vi "FTW-CodeGen-GenerateCode.vi"(0 "State In":T2, 5 "XRef":refnum<vi>, 7 "Terms":T1(array[cluster]), 9 "Diagram":refnum<vi>) -> (4 "State Out":T2, 6 "Reply":string[](array[string]), 8 "Generated Code?":bool)   [LabVIEW 2015, in "FTW-SQLite-Insert.xnode"]
uses:
  FTW-SQLite-Insert.xnode
  FTW-CodeGen-State.ctl
  FTW-CodeGen-XNodeCommonState.ctl
  FTW-CodeGen-XNodeReplyType.ctl
panel:
  # "Inputs"
  # "Outputs"
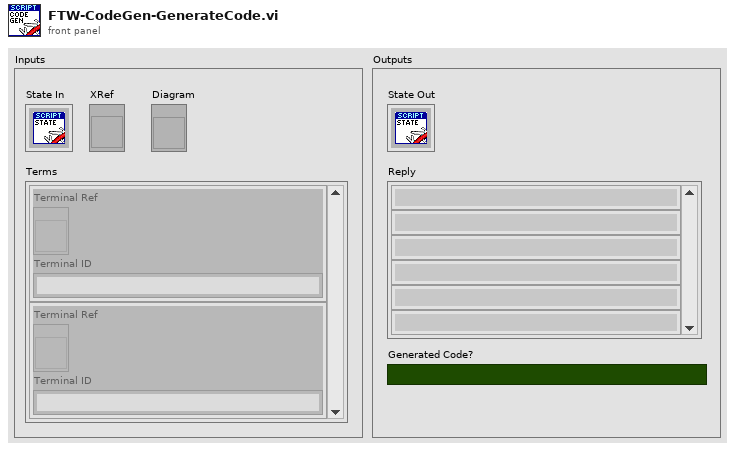
[diagram p1: front panel]
types:
  T1 = cluster{"Terminal Ref":refnum<vi>, "Terminal ID":string}[]
  T2 = typedef "FTW-SQLite-Insert.xnode/FTW-CodeGen-State.ctl" = cluster{"Cache":T3}
  T3 = typedef "FTW-CodeGen-XNodeCommonState.ctl" = cluster{"Terms":cluster{"Name":string, "Id":string, "Type":variant, "Bounds":cluster{"Left":i32, "Top":i32, "Right":i32, "Bottom":i32}, "Input?":bool, "Required?":bool, "Recommended?":bool, "Adaptive?":bool, "Hidden?":bool, "Direction":enum32{"Auto", "Up", "Down", "Left", "Right", "Center"}, "Break Wire?":bool, "English Name":string}[], "AdaptiveTerms":string[], "AdaptedTypes":variant[], "ForceCodeRegeneration?":bool, "LastGeneration":timestamp, "Errors":string[]}
  T4 = typedef "FTW-CodeGen-XNodeReplyType.ctl" = enum16{"UpdateState", "AdaptToInputs", "AdaptAndAugment", "CosmeticUpdate", "NoReply"}
  T5 = typedef "FTW-Reflection-Types.ctl" = enum16{"Unknown", "Void", "Array", "Cluster", "LVObject", "Boolean", "I8", "I16", "I32", "I64", "U8", "U16", "U32", "U64", "SGL", "DBL", "EXT", "CSG", "CDB", "CXT", "FXP", "EnumU8", "EnumU16", "EnumU32", "EnumU64", "SGLwithUnit", "DBLwithUnit", "EXTwithUnit", "CSGwithUnit", "CDBwithUnit", "CXTwithUnit", "String", "Path", "Picture", "Tag", "LVVariant", "Timestamp", "WaveformI8", "WaveformI16", "WaveformI32", "WaveformI64", "WaveformU8", "WaveformU16", "WaveformU32", "WaveformU64", "WaveformSGL", "WaveformDBL", "WaveformEXT", "WaveformCSG", "WaveformCDB", "WaveformCXT", "WaveformDigital", "WaveformUnknownType", "DigitalData", "DynamicData", "ExternalData", "FileByteStream", "TDMStream", "dotNET", "ActiveX", "VIServerReference", "VIReference", "ApplicationInstance", "Menu", "ConnectionDataSocket", "ConnectionVISA", "ConnectionBluetooth", "ConnectionIrDA", "ConnectionTCP", "ConnectionUDP", "ConnectionHTTPClient", "ConnectionFTP", "Occurrence", "Notifier", "Queue", "Rendezvous", "Semaphore", "RTFIFO", "EventPublisher", "EventRegistration", "EventCallback", "DataValueReference", "GenericClass", "GenericClassTag", "GenericClassDeepCopy", "GenericClassFlattened", "GenericClassTagFlattened", "GenericReferenceType", "WindowsRegistry", "OverloadedDatalogRef", "ReferenceUnknownType", "ByteArray", "ConPaneInterface", "FTWObject"}
  T6 = cluster{"Element Name":string, "Element Type":T5, "Element Value":variant}[]
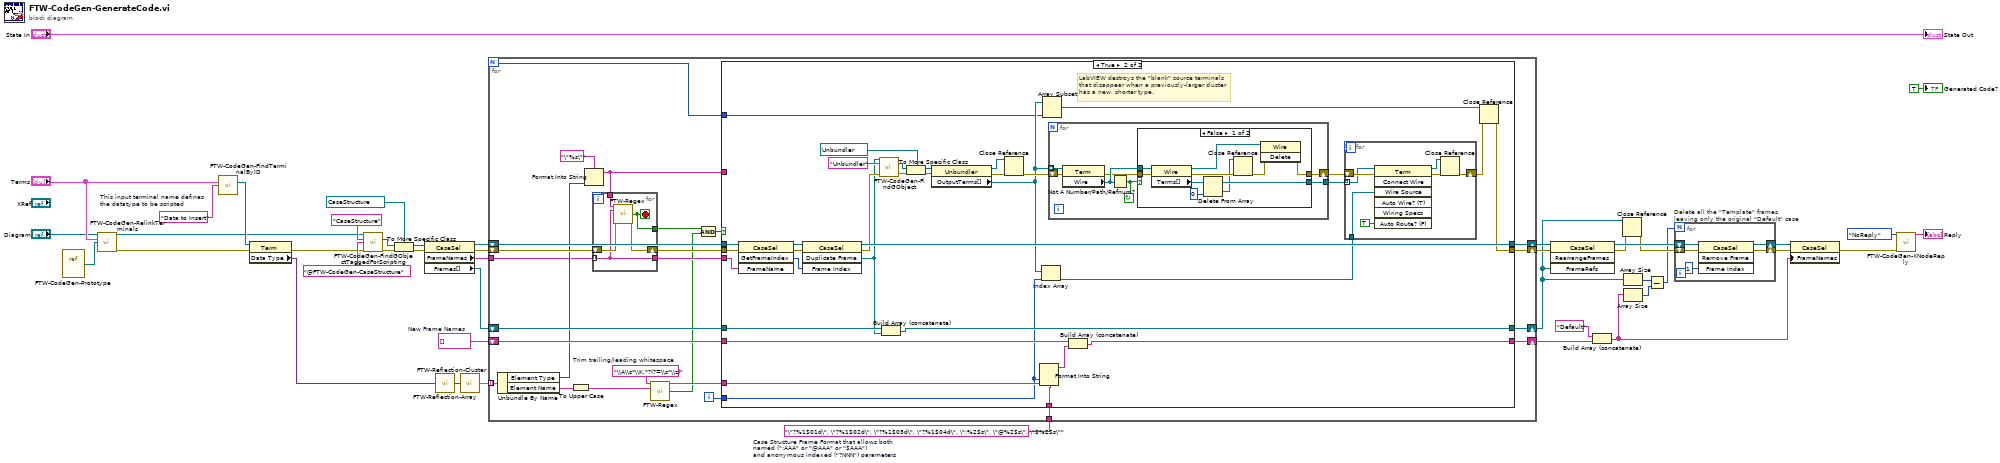
[diagram p0: block diagram]
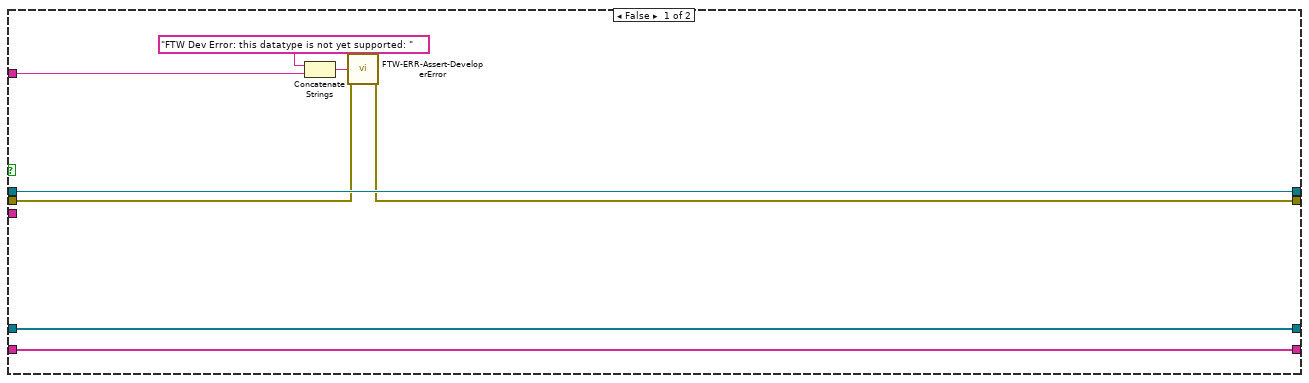
[diagram p2: hidden frame]
diagram:
  w13 = "\"?%1$01d\", \"?%1$02d\", \"?%1$03d\", \"?%1$04d\", \":%2$s\", \"@%2$s\", \"$%2$s\""  # Case Structure Frame Format that allows both named (":AAA" or "@AAA" or "$AAA") and anonymous indexed ("?NNN") parameters
  w1 = string[] []  # New Frame Names
  w4 = "Data to Insert"  # This input terminal name defines the datatype to be scripted
  n1 = vi-ref "FTW-CodeGen-Prototype.vi"() -> (w7:refnum<vi>)
  n2 = call "FTW-CodeGen-RelinkTerminals.vi"("Diagram"="Diagram", "Terms"="Terms", "PrototypeVI"=w7) -> ("Diagram out"=w2:refnum<vi>, "error out"=w10:errorcluster)  [unwired: 11 in]
  n3 = call "FTW-CodeGen-FindTerminalByID.vi"("Terms"="Terms", "Terminal ID"=w4) -> ("Terminal Ref"=w6:refnum<vi>)  [unwired: 12 in, 1 out]
  n4 = property class="Term"(reference=w6, error in=w10) -> (error out=w9:errorcluster, "Data Type"=w15:variant)  [unwired: 1 out]
  n5 = call "FTW-CodeGen-FindGObjectTaggedForScripting.vi"("GObject to Traverse"=w2, "Class Name"="CaseStructure", "Label Prefix to uniquely identify node"="@FTW-CodeGen-CaseStructure" ("Label to uniquely identify node"), "error in"=w9) -> ("GObject"=w40:refnum<vi>, "error out"=w39:errorcluster)  [unwired: 9 in, 1 out]
  n6 = To More Specific Class(target class=refnum<vi> refnum ("Object"), reference=w40, error in=w39) -> (specific class reference=w36:refnum<vi>, error out=w34:errorcluster)
  n7 = property class="CaseSel"(reference=w36, error in=w34) -> (reference out=w35:refnum<vi>, error out=w33:errorcluster, "FrameNames"=w32:string[], "Frames[]"=w21:refnum<vi>[])
  n8 = call "FTW-Reflection-Array.vi"("Array"=w15) -> ("Default Array Element"=w14:variant)  [unwired: 13 in, 1 out]
  n9 = call "FTW-Reflection-Cluster.vi"("Cluster"=w14) -> ("Cluster Elements"=w37:T6)  [unwired: 14 in]
  n10 = for {
    N -> [w44]
    tunnel: w37 -> [w66] mode=indexing
    tunnel: w32 -> [w52]
    shift-right: [w61] -> w26
    shift-left: w35 -> [w68]
    shift-right: [w62] -> w24
    shift-left: w33 -> [w67]
    shift-right: [w60] -> w20
    shift-left: w21 -> [w63]
    shift-right: [w58] -> w27
    shift-left: w1 -> [w59]
    tunnel: w13 -> [w54]
    i -> [w55]
    w48 = "\\A\\s*\\K.*?(?=\\s*\\z)"  # Trim trailing/leading whitespace
    n11 = Unbundle By Name(w66) -> ("Element Type"=w56:T5, "Element Name"=w57:string)
    n12 = To Upper Case(1:w57) -> (0:w50:string)
    n13 = Format Into String(format string="\"%s\"", w56) -> (resulting string=w64:string)  [unwired: 2 in, 1 out]
    n14 = for {
      tunnel: w64 -> [w72]
      shift-right: [w71] -> w53
      shift-left: w67 -> [w73]
      tunnel: w52 -> [w69] mode=indexing
      tunnel: [w70] -> w47
      tunnel: [w69] -> w51
      stop <- w70 stop-if-true
      n15 = call "FTW-Regex.vi"("Regular Expression"=w72, "Input String"=w69, "error in"=w73) -> ("Match Found?"=w70:bool, "error out"=w71:errorcluster)  [unwired: 8 in, 3 out]
    }
    n16 = call "FTW-Regex.vi"("Regular Expression"=w48, "Input String"=w50) -> ("Match"=w49:string, "Match Found?"=w45:bool)  [unwired: 9 in, 3 out]
    n17 = Compound Arithmetic op=AND(w47, w45) -> (w46:bool)
    n18 = case shown="True" w46 {
      tunnel: w53 -> [w75 w110]
      tunnel: w68 -> [w81 w111]
      tunnel: w63 -> [w80 w115]
      tunnel: [w80 w112] -> w60
      tunnel: [w74 w89] -> w62
      tunnel: [w81 w105] -> w61
      tunnel: w59 -> [w79 w114]
      tunnel: [w79 w113] -> w58
      tunnel: w51 -> [_ w106]
      tunnel: w49 -> [_ w88]
      tunnel: w55 -> [_ w87]
      tunnel: w64 -> [w77 _]
      tunnel: w54 -> [_ w86]
      tunnel: w44 -> [_ w83]
      frame False {
        n19 = Concatenate Strings("FTW Dev Error: this datatype is not yet supported: " ("Reason this error should never happen"), w77) -> (w76:string)
        n20 = call "FTW-ERR-Assert-DeveloperError.vi"("Reason this error should never happen"=w76, "error in"=w75) -> ("error out"=w74:errorcluster)  [unwired: 13 in]
      }
      frame True {
        # "LabVIEW destroys the \"blank\" source terminals\nthat disappear when a previously-larger cluster\nhas a new, shorter type."
        n21 = invoke class="CaseSel" method="GetFrameIndex"(reference=w111, error in=w110, "FrameName"=w106) -> (reference out=w109:refnum<vi>, error out=w108:errorcluster, "GetFrameIndex"=w107:i32)  [unwired: 1 in, 1 out]
        n22 = invoke class="CaseSel" method="Duplicate Frame"(reference=w109, error in=w108, "Frame Index"=w107) -> (reference out=w105:refnum<vi>, error out=w91:errorcluster, "Duplicate Frame"=w90:refnum<vi>)  [unwired: 1 in, 1 out]
        n23 = call "FTW-CodeGen-FindGObject.vi"("GObject to Traverse"=w90, "Class Name"="Unbundler", "error in"=w91) -> ("GObject"=w101:refnum<vi>, "error out"=w102:errorcluster)  [unwired: 11 in]
        n24 = Build Array (concatenate)(w115, w90) -> (w112:refnum<vi>[])
        n25 = To More Specific Class(target class=refnum<vi> refnum ("Object"), reference=w101, error in=w102) -> (specific class reference=w99:refnum<vi>, error out=w98:errorcluster)
        n26 = property class="Unbundler"(reference=w99, error in=w98) -> (reference out=w93:refnum<vi>, error out=w95:errorcluster, "OutputTerms[]"=w84:refnum<vi>[])
        n27 = Close Reference(reference=w93, error in (no error)=w95) -> (error out=w94:errorcluster)
        n28 = Format Into String(format string=w86, w87, w88) -> (resulting string=w104:string)  [unwired: 2 in, 1 out]
        n29 = Index Array(array=w84, index=w87) -> (element=w97:refnum<vi>)
        n30 = Array Subset(array=w84, length=w83) -> (w82:refnum<vi>[])  [unwired: 1 in]
        n31 = for {
          tunnel: w84 -> [w129] mode=indexing
          tunnel: [w126] -> w85
          shift-right: [w123] -> w96
          shift-left: w94 -> [w124]
          stop <- w127 continue-if-true
          n32 = property class="Term"(reference=w129, error in=w124) -> (error out=w125:errorcluster, "Wire"=w128:refnum<vi>)  [unwired: 1 out]
          n33 = Not A Number/Path/Refnum?(number/path/refnum=w128) -> (NaN/Path/Refnum?=w127:bool)
          n34 = case shown="False" w127 {
            tunnel: w128 -> [w139 _]
            tunnel: [w137 _] -> w126
            tunnel: w125 -> [w136 w140]
            tunnel: [w134 w140] -> w123
            frame False {
              n35 = property class="Wire"(reference=w139, error in=w136) -> (reference out=w135:refnum<vi>, error out=w133:errorcluster, "Terms[]"=w138:refnum<vi>[])
              n36 = Delete From Array(array=w138, index=0) -> (deleted portion=w131:refnum<vi>, array with subset deleted=w137:refnum<vi>[])  [unwired: 1 in]
              n37 = Close Reference(reference=w131, error in (no error)=w133) -> (error out=w132:errorcluster)
              n38 = invoke class="Wire" method="Delete"(reference=w135, error in=w132) -> (error out=w134:errorcluster)  [unwired: 1 in, 2 out]
            }
            frame True {
            }
          }
        }
        n39 = Build Array (concatenate)(w114, w104) -> (w113:string[])
        n40 = for {
          tunnel: w97 -> [w122]
          shift-right: [w116] -> w92
          shift-left: w96 -> [w120]
          tunnel: w85 -> [w119] mode=indexing
          n41 = invoke class="Term" method="Connect Wire"(reference=w119, error in=w120, "Wire Source"=w122, "Auto Route? (F)"=TRUE) -> (reference out=w118:refnum<vi>, error out=w117:errorcluster)  [unwired: 3 in, 5 out]
          n42 = Close Reference(reference=w118, error in (no error)=w117) -> (error out=w116:errorcluster)
        }
        n43 = Close Reference(reference=w82, error in (no error)=w92) -> (error out=w89:errorcluster)
      }
    }
  }
  n44 = invoke class="CaseSel" method="RearrangeFrames"(reference=w26, error in=w24, "FrameRefs"=w20) -> (reference out=w25:refnum<vi>, error out=w23:errorcluster)  [unwired: 1 in, 2 out]
  n45 = Build Array (concatenate)("Default", w27) -> (w19:string[])
  n46 = Close Reference(reference=w20, error in (no error)=w23) -> (error out=w22:errorcluster)
  n47 = Array Size(array=w20) -> (size(s)=w18:i32)
  n48 = Array Size(array=w19) -> (size(s)=w17:i32)
  n49 = Subtract(x=w18, y=w17) -> (x-y=w16:i32)
  n50 = for "Delete all the \"Template\" frames,\nleaving only the original \"Default\" case" {
    N: w16 -> [_]
    shift-right: [w142] -> w30
    shift-left: w22 -> [w143]
    shift-right: [w144] -> w31
    shift-left: w25 -> [w145]
    n51 = invoke class="CaseSel" method="Remove Frame"(reference=w145, error in=w143, "Frame Index"=u32 1) -> (reference out=w144:refnum<vi>, error out=w142:errorcluster)  [unwired: 1 in, 2 out]
  }
  n52 = property class="CaseSel"(reference=w31, error in=w30, "FrameNames"=w19) -> (error out=w12:errorcluster)  [unwired: 1 out]
  n53 = call "FTW-CodeGen-XNodeReply.vi"("XNode Reply Type"=FTW-CodeGen-XNodeReplyType."NoReply", "error in"=w12) -> ("Reply"=→"Reply":string[])  [unwired: 13 in]
  "State Out" <- "State In"
  "Generated Code?" <- TRUE ("Generated Code?")
